vi "Find Center.vi"(5 "Position":i32, 7 "Tray Number":dbl format="%#_13g", 8 "Type of Hexaboard":T1, 9 "XYZTheta":dbl[](array[numeric]), 11 "Gantry In":refnum<k24>) -> (1 "XYZTheta Centers":dbl[][](array[numeric]), 3 "Gantry Out":refnum<k24>)   [LabVIEW 2021, in "Assembly Tray.lvclass"]
uses:
  Assembly Tray.lvclass
  Find Tray.ctl
  Controller/Camera/Machine Vision.ctl
  C:/Program Files (x86)/Aerotech/A3200/LabVIEW/2010/Bin/Aerotech.A3200.dll
  Program Files (x86)/Aerotech/A3200/LabVIEW/2010/Bin/Aerotech.A3200.dll
  Controller/Camera/Image processing.ctl
  Controller/Camera/Camera settings.ctl
  Controller/Camera/Material.ctl
  Routine/TypeOfHexaboard.ctl
  Program Files (x86)/National Instruments/LabVIEW 2021/examples/Connectivity/Python/support/PythonVersionsEnum.ctl
  Controller/Camera/Camera.lvclass
  Controller/Motion/A3200/A3200.lvclass
  Controller/Motion/Motion.lvclass
  Routine/Routine.lvclass
panel:
  out "Move by":dbl[](array[numeric])
  in  "Autofiducial (Beta)":bool
  in  "Focus step size":dbl format="%#_13g"
  in  "number of focus steps":i32
  out "Average Strength":dbl
  in  "Focus":bool
  in  "Material":T2
  in  "Camera settings":T3={"Gamma"=1.6, "Gain"=0, "Sharpness"=0, "Contrast"=0.0, "Exposure"=0.0078125} {"Exposure" min=0.000244140625 max=0.5 scale=0.0002..0.5; "Contrast" min=0.0 max=1.0 scale=0.001..1.0; "Sharpness" min=0 max=2 step=1 scale=0.0..2.0; "Gain" min=0 max=100 step=1 scale=0.1..100.0; "Gamma" min=0.01 max=10.0 scale=0.01..10.0}
  in  "Image processing":T4={"Brightness"=128.0, "Contrast"=45.0, "Gamma"=1.0471123} {"Brightness" scale=0.0..400.0; "Contrast" scale=0.0..90.0; "Gamma" scale=0.005..5.0}
  in  "Override presets":bool
  out "Both fiducials recorded":bool
  in  "Machine Vision":T5
  out "Right Fiducial":dbl[](array[numeric]) format="%.6g"
  out "Left Fiducial":dbl[](array[numeric]) format="%.6g"
  out "Gantry":dbl[](array[numeric]) format="%.6g"
  out "Sum":dbl[](array[numeric]) format="%.6g"
  out "Camera":dbl[](array[numeric]) format="%.6g"
  in  "Carrier Tray":T6
  out "Image":T7(plugin-control)
  out "Center":dbl[](array[numeric]) format="%.6g"
  in  "Position Number":i16
  in  "Go to Center":bool
  in  "Calculate":bool
  in  "Record Bottom":bool
  in  "Record Top":bool
  in  "Go to Bottom Fiducial":bool
  in  "Go to Top Fiducial":bool
  in  "Joystick":bool
  in  "Stop":bool
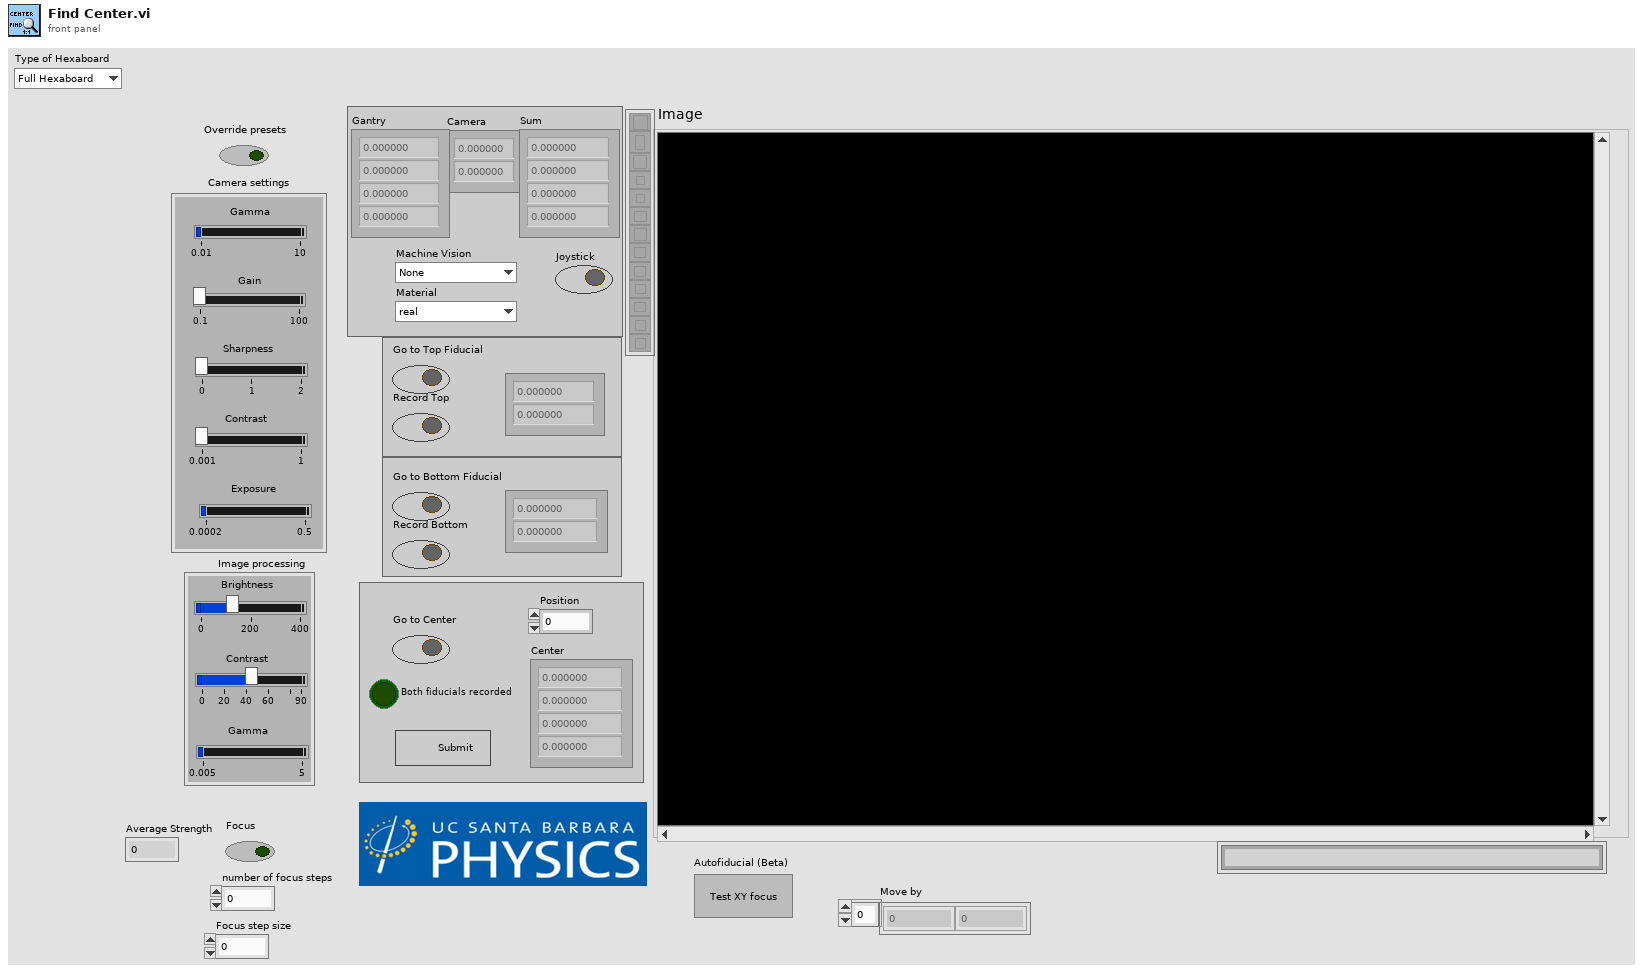
[diagram p1: front panel]
types:
  T1 = typedef "Routine.lvclass/TypeOfHexaboard.ctl" = enum16{"Full Hexaboard", "Right Partial PCB", "Right Partial Sensor", "Al Dummy Right Partial Sensor"}
  T2 = typedef "Camera.lvclass/Material.ctl" = enum16{"real", "dummy", "PETG"}
  T3 = typedef "Camera.lvclass/Camera settings.ctl" = cluster{"Gamma":dbl, "Gain":i64, "Sharpness":i64, "Contrast":dbl, "Exposure":dbl}
  T4 = typedef "Camera.lvclass/Image processing.ctl" = cluster{"Brightness":sgl, "Contrast":sgl, "Gamma":sgl}
  T5 = typedef "Camera.lvclass/Machine Vision.ctl" = enum16{"None", "Tray Fiducials", "Sensor Fiducials", "HPK Silicon", "Partial Hexaboard", "Partial Hexaboard Test", "100um dot", "Hexaboard", "Corner (TL, BR)", "Corner (BL, TR)", "V3 Sensor Cross", "V3 Sensor Circle"}
  T6 = typedef "Assembly Tray.lvclass/Find Tray.ctl" = cluster{"Gantry Fiducials":dbl[], "Relative Coordinates":dbl[][], "Camera Fiducials":dbl[][], "XYZTheta Centers":dbl[][], "Workspace Center":dbl[], "Syringe Relative Coordinates":dbl[], "Gantry Region":dbl, "Fiducials":path, "New Fiducials":dbl[][], "Past Fiducials":dbl[][], "XYZTheta":dbl[], "Position":dbl}
  T7 = typedef "IMAQ Image.ctl" = refnum<image>
  T8 = typedef "PythonVersionsEnum.ctl" = enum16{"3.6", "3.7", "3.8", "3.9"}
  T9 = typedef "File Paths.ctl" = cluster{"Glue Pattern Folder":path, "Carrier Tray Folder":path, "Pick Up Tool Fixture Folder":path, "Components Folder":path, "Bellows Tool Offset.txt":path, "Pick Up Tool Offset.txt":path, "Dispense Tip Offset.txt":path, "Log Files":path, "Gantry Assembly Map.txt":path, "Syringe and offset map.txt":path}
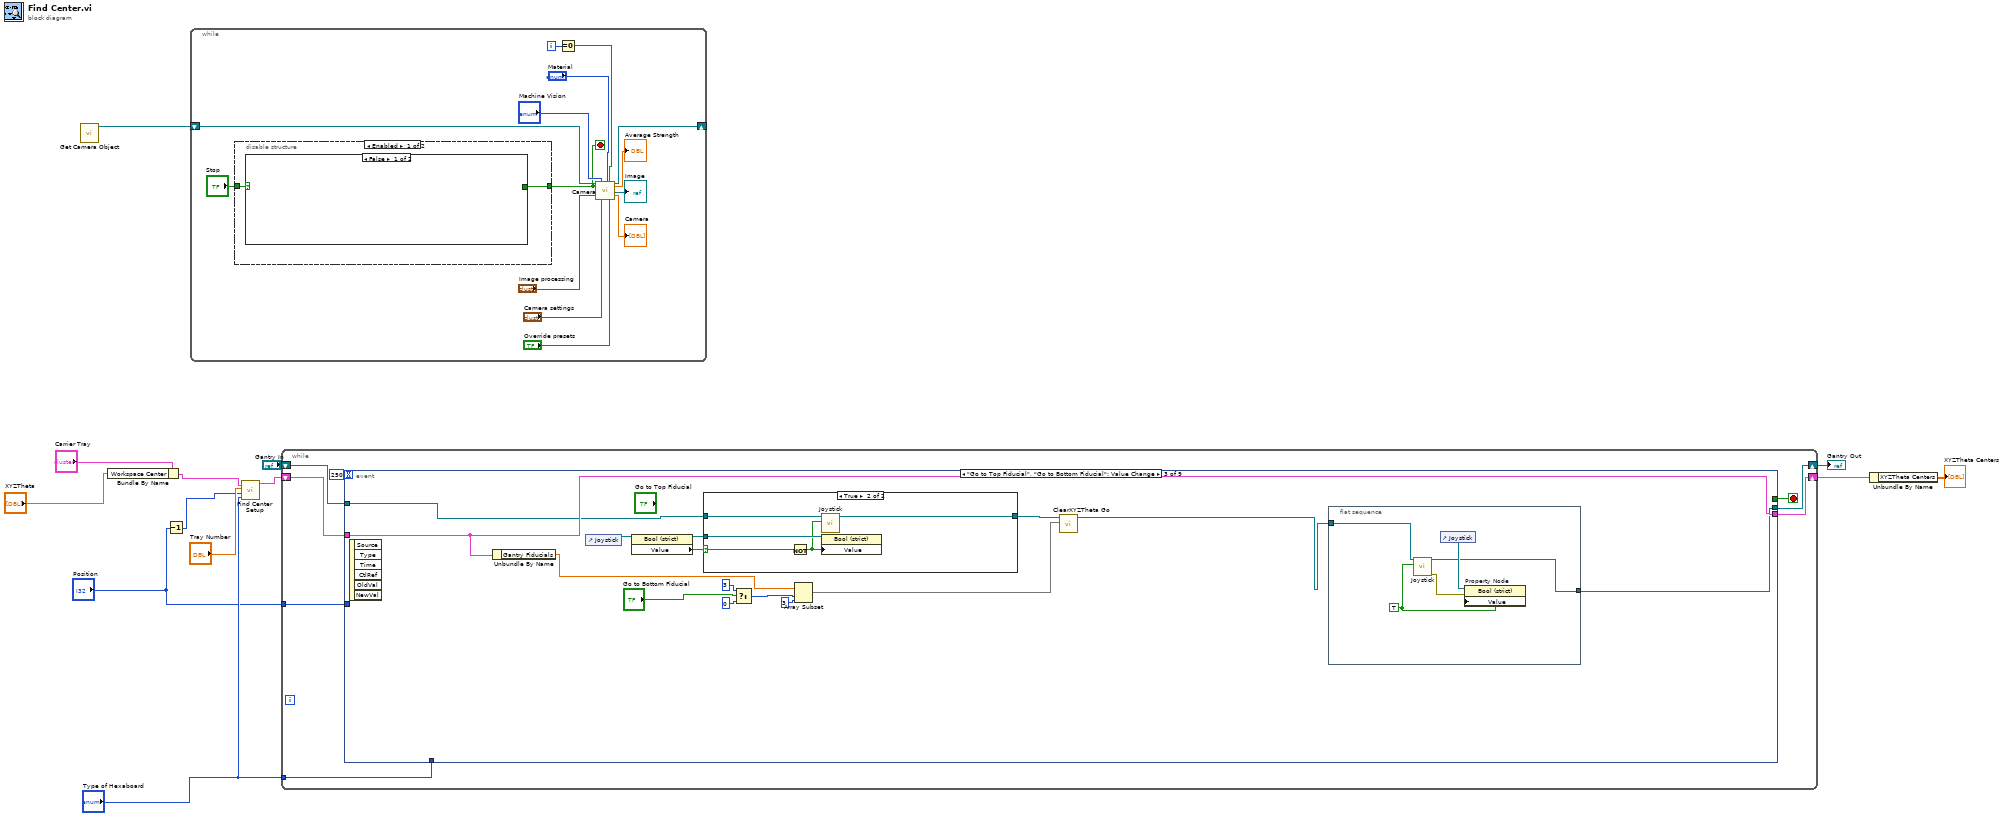
[diagram p0: block diagram]
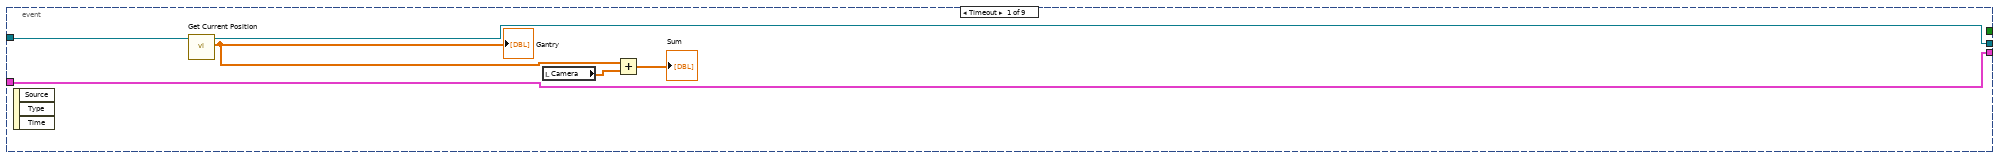
[diagram p2: hidden frame]
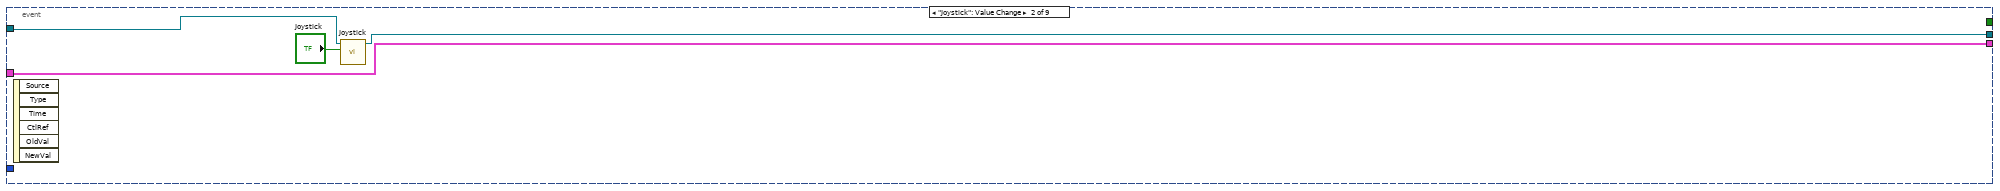
[diagram p3: hidden frame]
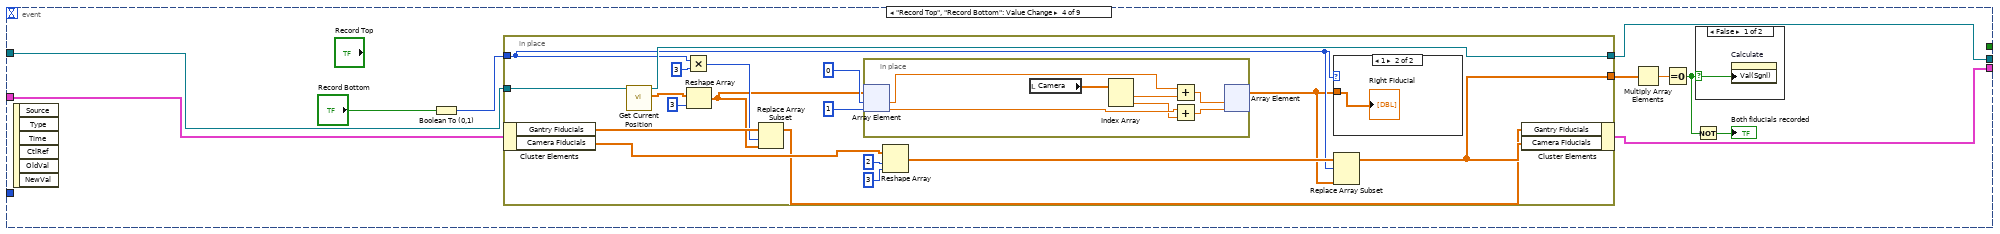
[diagram p5: hidden frame]
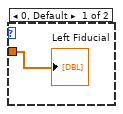
[diagram p7: hidden frame]
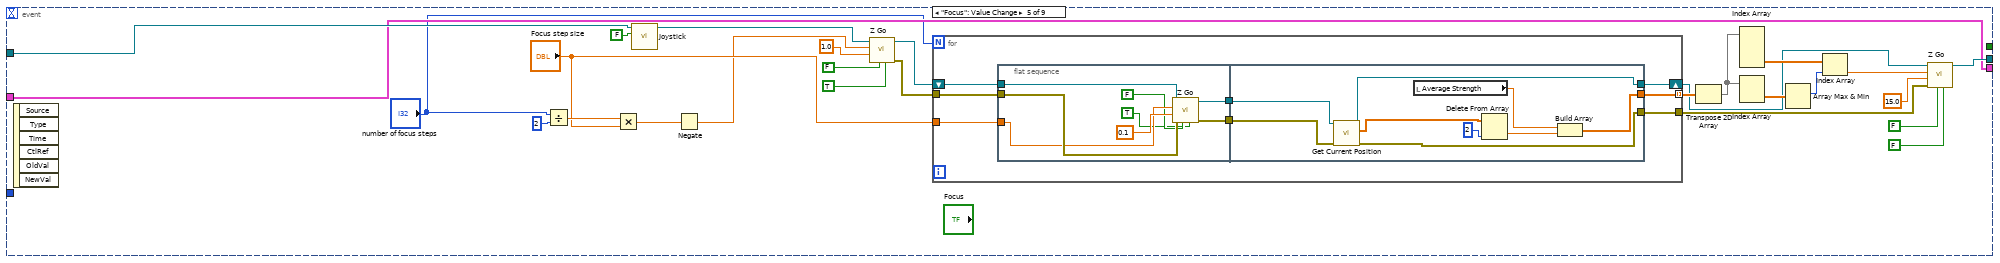
[diagram p8: hidden frame]
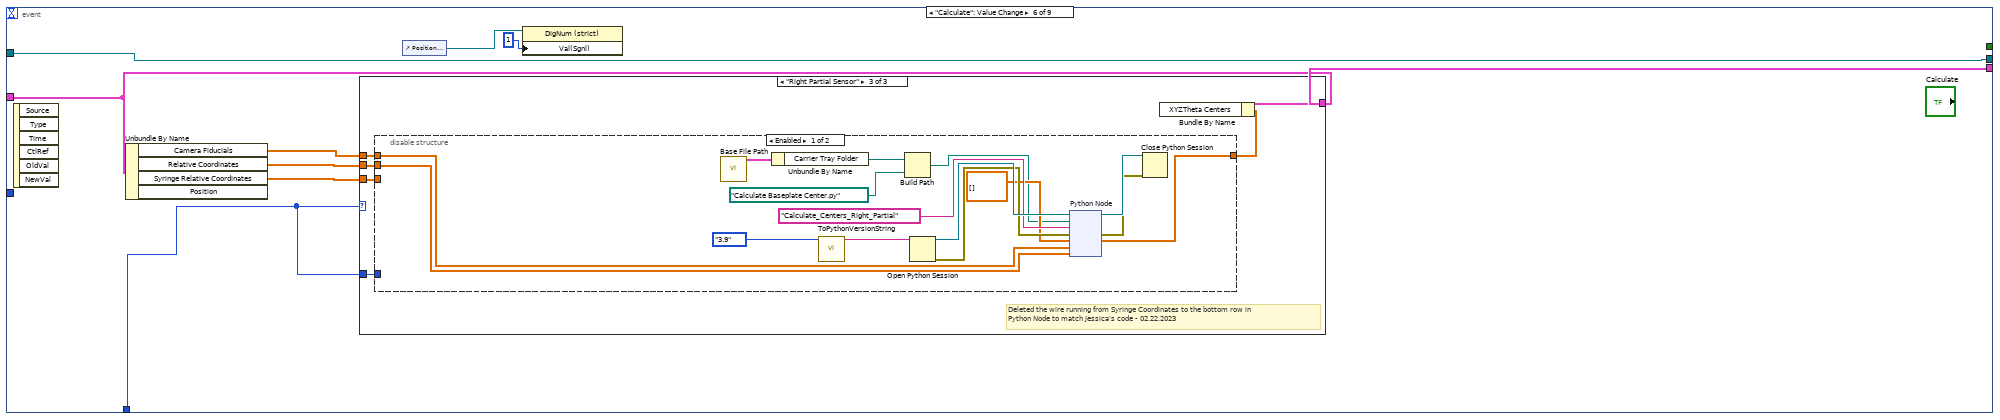
[diagram p9: hidden frame]
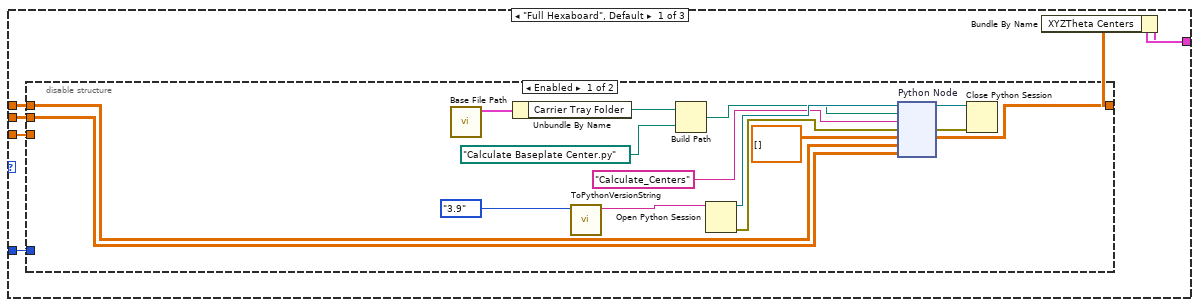
[diagram p10: hidden frame]
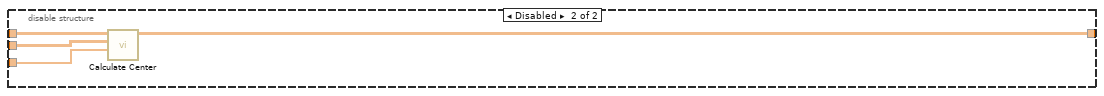
[diagram p11: hidden frame]
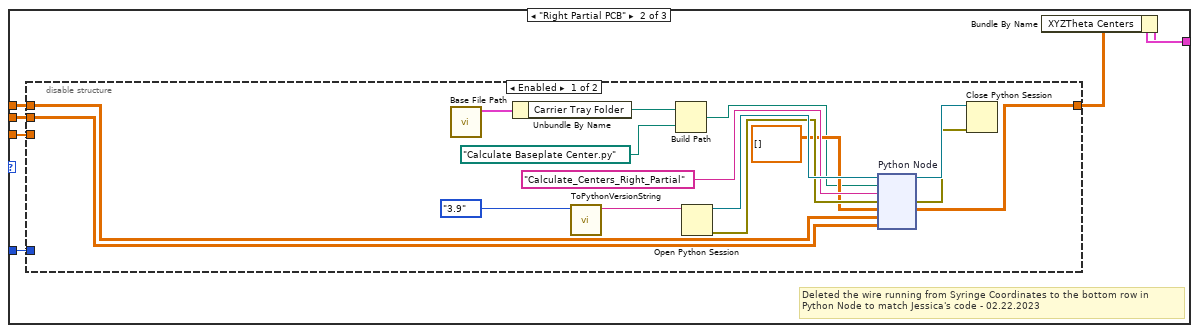
[diagram p12: hidden frame]
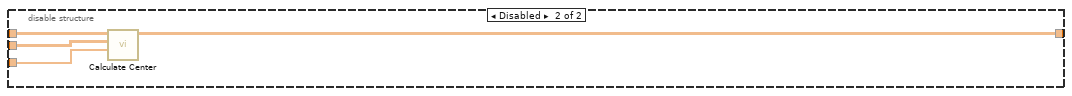
[diagram p13: hidden frame]
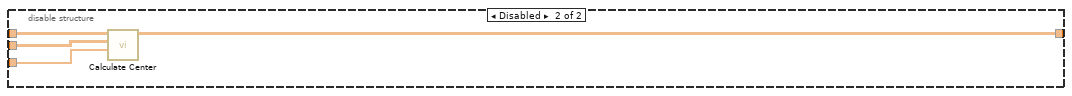
[diagram p14: hidden frame]
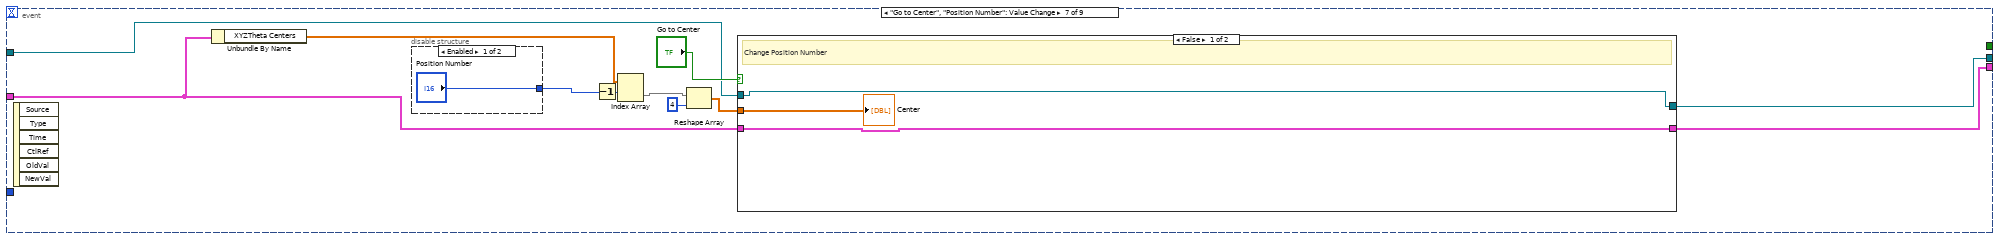
[diagram p15: hidden frame]
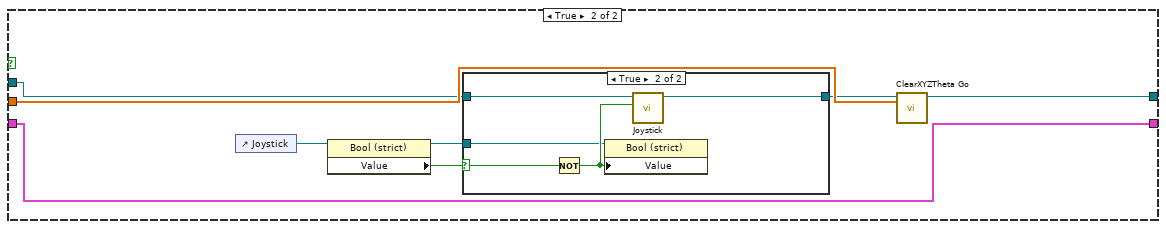
[diagram p17: hidden frame]
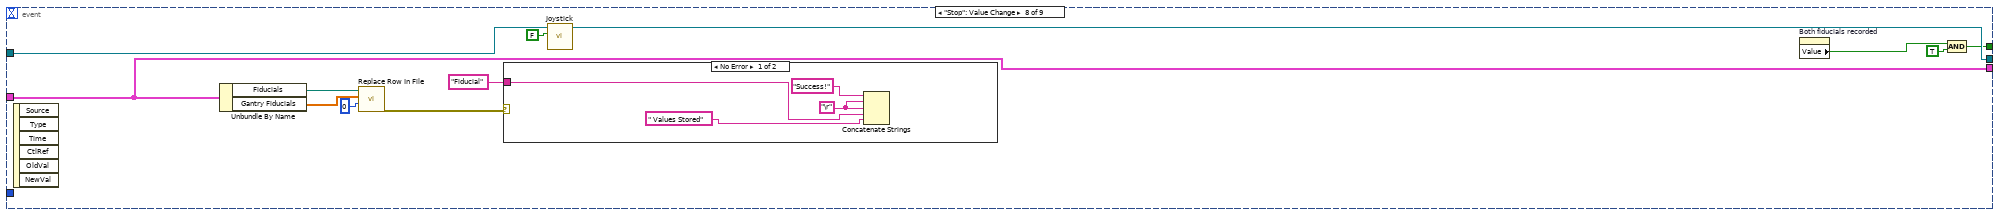
[diagram p19: hidden frame]
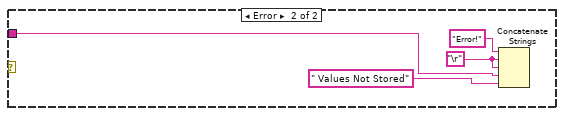
[diagram p20: hidden frame]
diagram:
  n1 = call "Get Camera Object.vi"() -> ("Camera out"=w6:refnum<class "Camera.lvclass">)  [unwired: 10 in, 1 out]
  n2 = Bundle By Name(cluster="Carrier Tray", "Workspace Center"="XYZTheta") -> (w10:T6)
  n3 = Decrement(x="Position") -> (x-1=w3:i32)
  n4 = while {
    shift-right: [w23] -> _
    shift-left: w6 -> [w27]
    i -> [w17]
    stop <- w22 stop-if-true
    n5 = disable-structure shown="Enabled" {
      disable-tunnel: [w28 w35] -> w22
      disable-tunnel: "Stop" -> [w29 w35]
      frame Enabled {
        n6 = case shown="False" w29 {
          tunnel: [_ w30] -> w28
          frame False {
          }
          frame True {
            n7 = property on="Both fiducials recorded" class="Bool (strict)"() -> ("Value"=w31:bool)  [unwired: 2 in, 2 out]
            n8 = case shown="False" w31 {
              tunnel: [_ TRUE] -> w30
              frame False {
                n9 = One Button Dialog(message="Atleast one fiducial not recorded!") -> ()  [unwired: 1 in, 1 out]
              }
              frame True {
                n10 = property on="Both fiducials recorded" class="Bool (strict)"("Val(Sgnl)"=FALSE) -> ()  [unwired: 2 in, 2 out]
              }
            }
          }
        }
      }
      frame Disabled {
      }
    }
    n11 = Equal To 0?(x=w17) -> (x = 0?=w16:bool)
    n12 = call "Camera.vi"("Camera in"=w27, "Stop"=w22, "BCG Image Processing"="Image processing", "Machine Vision"="Machine Vision", "Camera settings"="Camera settings", "Material"="Material", "Loop 0"=w16, "Override presets"="Override presets") -> ("Camera out"=w23:refnum<class "Camera.lvclass">, "Average Strength"=→"Average Strength":dbl, "Image"=→"Image":T7, "Camera"=→"Camera":dbl[])  [unwired: 5 in, 3 out]
  }
  n13 = call "Find Center Setup.vi"("Carrier Tray"=w10, "Tray Number"="Tray Number", "Position"=w3, "Type of Hexaboard"="Type of Hexaboard") -> ("Assembly Tray Out"=w13:T6)  [unwired: 6 in]
  n14 = while {
    shift-right: [w42] -> w12
    shift-left: w13 -> [w43]
    shift-right: [w38] -> w4
    shift-left: "Gantry In" -> [w39]
    tunnel: "Type of Hexaboard" -> [w37]
    tunnel: "Position" -> [w36]
    stop <- w41 stop-if-true
    n15 = event shown="[2] \"Go to Top Fiducial\", \"Go to Bottom Fiducial\": Value Change" {
      selector: _ -> [_ _ _ _ _ _ _ _ _]
      dyn-events: _ -> [_ _ _ _ _ _ _ _ _]
      timeout: 250 -> [_ _ _ _ _ _ _ _ _]
      tunnel: [w47 w53 w68 w89 w129 w176 w266 w293 w306] -> w42
      tunnel: w43 -> [w47 w53 w68 w84 w129 w170 w267 w293 w306]
      tunnel: [_ _ _ _ _ _ _ w288 _] -> w41
      tunnel: w39 -> [w46 w52 w60 w83 w131 w175 w264 w294 w308]
      tunnel: [w44 w50 w55 w82 w130 w175 w260 w289 w309] -> w38
      tunnel: w37 -> [_ _ _ _ _ w171 _ _ _]
      tunnel: w36 -> [_ _ _ _ _ _ _ _ _]
      event Timeout {
        n16 = event-data() -> ()  [unwired: 1 in, 3 out]
        n17 = call "Get Current Position.vi"("Gantry In"=w46) -> ("XYZTheta Out"=w45:dbl[], "Gantry Out"=w44:refnum<k24>)  [unwired: 8 in, 1 out]
        "Gantry" <- w45
        n18 = local read "Camera"() -> (w49:dbl[])
        n19 = Add(x=w45, y=w49) -> (x+y=→"Sum":dbl[])
      }
      event "Joystick": Value Change {
        n20 = event-data() -> ()  [unwired: 1 in, 6 out]
        n21 = call "Joystick.vi"("Joystick"="Joystick", "Gantry In"=w52) -> ("Gantry Out"=w50:refnum<k24>)  [unwired: 8 in, 1 out]
      }
      event "Go to Top Fiducial", "Go to Bottom Fiducial": Value Change {
        n22 = event-data() -> ()  [unwired: 1 in, 6 out]
        n23 = Unbundle By Name "Unbundle By Name"(w68) -> ("Gantry Fiducials"=w57:dbl[])
        n24 = control-ref of="Joystick"() -> (w67:refnum<vi>)
        n25 = property class="Bool (strict)"(reference=w67) -> (reference out=w58:refnum<vi>, "Value"=w61:bool)  [unwired: 1 in, 1 out]
        n26 = case shown="True" w61 {
          selector: w61 -> [_ w79]
          tunnel: w60 -> [w74 w77]
          tunnel: [w74 w76] -> w59
          tunnel: w58 -> [_ w78]
          frame False {
          }
          frame True {
            n27 = Not(x=w79) -> (.not. x?=w75:bool)
            n28 = call "Joystick.vi"("Joystick"=w75, "Gantry In"=w77) -> ("Gantry Out"=w76:refnum<k24>)  [unwired: 8 in, 1 out]
            n29 = property class="Bool (strict)"(reference=w78, "Value"=w75) -> ()  [unwired: 1 in, 2 out]
          }
        }
        n30 = Select(t=3, s="Go to Bottom Fiducial", f=0) -> (s? t:f=w65:i32)
        n31 = Array Subset "Array Subset"(array=w57, index=w65, length=3) -> (w56:dbl[])
        n32 = call "ClearXYZTheta Go.vi"("XYZTheta In"=w56, "Gantry In"=w59) -> ("Gantry Out"=w54:refnum<k24>)  [unwired: 7 in, 2 out]
        n33 = flat-sequence {
          tunnel: w54 -> [w73]
          tunnel: [w70] -> w55
          frame #0 {
            w69 = TRUE
            n34 = call "Joystick.vi"("Joystick"=w69, "Gantry In"=w73) -> ("error out"=w71:errorcluster, "Gantry Out"=w70:refnum<k24>)  [unwired: 8 in]
            n35 = control-ref of="Joystick"() -> (w72:refnum<vi>)
            n36 = property on="Property Node" class="Bool (strict)"(reference=w72, error in=w71, "Value"=w69) -> ()  [unwired: 2 out]
          }
        }
      }
      event "Record Top", "Record Bottom": Value Change {
        n37 = event-data() -> ()  [unwired: 1 in, 6 out]
        n38 = Boolean To (0,1)(Boolean="Record Bottom") -> (0, 1=w86:i16)
        n39 = in-place {
          in-place-border: [w102] -> w87
          in-place-border: w86 -> [w95]
          in-place-border: w83 -> [w97]
          in-place-border: [w96] -> w82
          n40 = in-place-cluster #1(w84) -> ("Gantry Fiducials"=w99:dbl[], "Camera Fiducials"=w106:dbl[][])
          n41 = call "Get Current Position.vi"("Gantry In"=w97) -> ("XYZTheta Out"=w100:dbl[], "Gantry Out"=w96:refnum<k24>)  [unwired: 8 in, 1 out]
          n42 = Multiply(x=w95, y=i16 3) -> (x*y=w93:i16)
          n43 = Reshape Array(w100, 3 ("dimension size")) -> (w92:dbl[])
          n44 = Replace Array Subset(array=w99, new element=w92, index=w93) -> (w98:dbl[])
          n45 = in-place {
            n46 = in-place-array #2(w92, 0, 1) -> (w114:dbl, w112:dbl)
            n47 = local read "Camera"() -> (w115:dbl[])
            n48 = Index Array(array=w115) -> (element #1=w113:dbl, element #2=w111:dbl)  [unwired: 2 in]
            n49 = Add(x=w114, y=w113) -> (x+y=w109:dbl)
            n50 = Add(x=w112, y=w111) -> (x+y=w110:dbl)
            n51 = in-place-array #2(w109, w110) -> (w91:dbl[])  [unwired: 2 out]
          }
          n52 = Reshape Array(w106, 2 ("length"), 3 ("dimension size")) -> (w105:dbl[][])
          n53 = case shown="1" w95 {
            tunnel: w91 -> [w116 w117]
            frame 0, Default {
              "Left Fiducial" <- w116
            }
            frame 1 {
              "Right Fiducial" <- w117
            }
          }
          n54 = Replace Array Subset(array=w105, new element=w91, index (row)=w95) -> (w102:dbl[][])  [unwired: 1 in]
          n55 = in-place-cluster #1("Gantry Fiducials"=w98, "Camera Fiducials"=w102) -> (w89:T6)
        }
        n56 = Multiply Array Elements(1:w87) -> (0:w88:dbl)
        n57 = Equal To 0?(x=w88) -> (x = 0?=w81:bool)
        n58 = Not(x=w81) -> (.not. x?=→"Both fiducials recorded":bool)
        n59 = case shown="False" w81 {
          selector: w81 -> [w90 _]
          frame False {
            n60 = property on="Calculate" class="Bool (strict)"("Val(Sgnl)"=w90) -> ()  [unwired: 2 in, 2 out]
          }
          frame True {
          }
        }
      }
      event "Focus": Value Change {
        n61 = event-data() -> ()  [unwired: 1 in, 6 out]
        n62 = Divide(x="number of focus steps", y=2) -> (x/y=w133:dbl)
        n63 = Multiply(x=w133, y="Focus step size") -> (x*y=w132:dbl)
        n64 = call "Joystick.vi"("Joystick"=FALSE, "Gantry In"=w131) -> ("Gantry Out"=w125:refnum<k24>)  [unwired: 8 in, 1 out]
        n65 = Negate(x=w132) -> (-x=w123:dbl)
        n66 = call "Z Go.vi"("Increment"=TRUE, "Return Immediately"=FALSE ("Increment"), "Speed In"=1.0 ("Speed"), "Position In"=w123, "Gantry In"=w125) -> ("error out"=w120:errorcluster, "Gantry Out"=w124:refnum<k24>)  [unwired: 3 in, 2 out]
        n67 = for {
          N: "number of focus steps" -> [_]
          tunnel: [w149] -> w143 mode=indexing
          tunnel: w120 -> [w148]
          tunnel: [w146] -> w136
          shift-right: [w150] -> w137
          shift-left: w124 -> [w152]
          tunnel: "Focus step size" -> [w145]
          n68 = flat-sequence {
            tunnel: w152 -> [w160]
            tunnel: [w159] -> w151
            tunnel: w148 -> [w157]
            tunnel: [w158] -> w147
            tunnel: w145 -> [w155]
            tunnel: w151 -> [w169]
            tunnel: [w168] -> w150
            tunnel: [w167] -> w149
            tunnel: w147 -> [w163]
            tunnel: [w162] -> w146
            frame #0 {
              n69 = call "Z Go.vi"("Increment"=TRUE, "Return Immediately"=FALSE ("Increment"), "error in (no error)"=w157, "Speed In"=0.1 ("Speed"), "Position In"=w155, "Gantry In"=w160) -> ("error out"=w158:errorcluster, "Gantry Out"=w159:refnum<k24>)  [unwired: 2 in, 2 out]
            }
            frame #1 {
              n70 = call "Get Current Position.vi"("error in (no error)"=w163, "Gantry In"=w169) -> ("error out"=w162:errorcluster, "XYZTheta Out"=w166:dbl[], "Gantry Out"=w168:refnum<k24>)  [unwired: 7 in]
              n71 = local read "Average Strength"() -> (w161:dbl)
              n72 = Delete From Array(array=w166, index=2) -> (deleted portion=w164:dbl)  [unwired: 1 in, 1 out]
              n73 = Build Array(w161, w164) -> (w167:dbl[])
            }
          }
        }
        n74 = Transpose 2D Array(2D array=w143) -> (transposed array=w142:dbl[][])
        n75 = Index Array(array=w142) -> (element #2=w141:dbl[])  [unwired: 4 in, 1 out]
        n76 = Index Array(array=w142) -> (element=w144:dbl[])  [unwired: 2 in]
        n77 = Array Max & Min(array=w144) -> (max index (indices)=w140:i32)  [unwired: 3 out]
        n78 = Index Array(array=w141, index=w140) -> (element=w139:dbl)
        n79 = call "Z Go.vi"("Increment"=FALSE, "Return Immediately"=FALSE ("Increment"), "error in (no error)"=w136, "Speed In"=15.0 ("Speed"), "Position In"=w139, "Gantry In"=w137) -> ("Gantry Out"=w130:refnum<k24>)  [unwired: 2 in, 3 out]
      }
      event "Calculate": Value Change {
        n80 = event-data() -> ()  [unwired: 1 in, 6 out]
        n81 = Unbundle By Name "Unbundle By Name"(w170) -> ("Camera Fiducials"=w172:dbl[][], "Relative Coordinates"=w173:dbl[][], "Syringe Relative Coordinates"=w174:dbl[])  [unwired: 1 out]
        n82 = case shown="\"Right Partial Sensor\"" w171 {
          tunnel: w170 -> [w185 w211 w237]
          tunnel: [w184 w210 w236] -> w176
          tunnel: w174 -> [w183 w209 w235]
          tunnel: w173 -> [w182 w208 w234]
          tunnel: w172 -> [w181 w207 w233]
          tunnel: w171 -> [w179 w205 w231]
          frame "Full Hexaboard", Default {
            n83 = disable-structure shown="Enabled" {
              disable-tunnel: w181 -> [w192 w203]
              disable-tunnel: w182 -> [w191 w202]
              disable-tunnel: w183 -> [_ w201]
              disable-tunnel: [w186 w204] -> w180
              disable-tunnel: w179 -> [_ _]
              frame Enabled {
                n84 = call "Base File Path.vi"() -> ("Paths Out"=w193:T9)  [unwired: 11 in]
                n85 = Unbundle By Name(w193) -> ("Carrier Tray Folder"=w189:path)
                n86 = call "ToPythonVersionString.vi"("python version"=PythonVersionsEnum."3.9") -> ("python version string"=w199:string)  [unwired: 10 in]
                n87 = Build Path(base path=w189, name or relative path=path "Calculate Baseplate Center.py") -> (appended path=w188:path)
                n88 = Open Python Session(python version=w199) -> (session out=w198:refnum<k35>, error out=w196:errorcluster)  [unwired: 2 in]
                n89 = node "Python Node"(w198, w188, "Calculate_Centers" ("function name"), w196, dbl[][] [], w192, w191) -> (w197:refnum<k35>, w195:errorcluster, w186:dbl[][])  [unwired: 2 in, 2 out]
                n90 = Close Python Session(session in=w197, error in=w195) -> ()  [unwired: 1 out]
              }
              frame Disabled {
                n91 = call "Calculate Center.vi"("Syringe Coordinates"=w201, "Relative Coordinates"=w202, "Fiducial Measurements"=w203) -> ("XYZTheta Centers"=w204:dbl[][])  [unwired: 8 in]
              }
            }
            n92 = Bundle By Name(cluster=w185, "XYZTheta Centers"=w180) -> (w184:T6)
          }
          frame "Right Partial PCB" {
            # "Deleted the wire running from Syringe Coordinates to the bottom row in\nPython Node to match Jessica's code - 02.22.2023"
            n93 = disable-structure shown="Enabled" {
              disable-tunnel: w207 -> [w218 w229]
              disable-tunnel: w208 -> [w217 w228]
              disable-tunnel: w209 -> [_ w227]
              disable-tunnel: [w212 w230] -> w206
              disable-tunnel: w205 -> [_ _]
              frame Enabled {
                n94 = call "Base File Path.vi"() -> ("Paths Out"=w219:T9)  [unwired: 11 in]
                n95 = Unbundle By Name(w219) -> ("Carrier Tray Folder"=w215:path)
                n96 = call "ToPythonVersionString.vi"("python version"=PythonVersionsEnum."3.9") -> ("python version string"=w225:string)  [unwired: 10 in]
                n97 = Build Path(base path=w215, name or relative path=path "Calculate Baseplate Center.py") -> (appended path=w214:path)
                n98 = Open Python Session(python version=w225) -> (session out=w224:refnum<k35>, error out=w222:errorcluster)  [unwired: 2 in]
                n99 = node "Python Node"(w224, w214, "Calculate_Centers_Right_Partial" ("function name"), w222, dbl[][] [], w218, w217) -> (w223:refnum<k35>, w221:errorcluster, w212:dbl[][])  [unwired: 2 in, 2 out]
                n100 = Close Python Session(session in=w223, error in=w221) -> ()  [unwired: 1 out]
              }
              frame Disabled {
                n101 = call "Calculate Center.vi"("Syringe Coordinates"=w227, "Relative Coordinates"=w228, "Fiducial Measurements"=w229) -> ("XYZTheta Centers"=w230:dbl[][])  [unwired: 8 in]
              }
            }
            n102 = Bundle By Name(cluster=w211, "XYZTheta Centers"=w206) -> (w210:T6)
          }
          frame "Right Partial Sensor" {
            # "Deleted the wire running from Syringe Coordinates to the bottom row in\nPython Node to match Jessica's code - 02.22.2023"
            n103 = disable-structure shown="Enabled" {
              disable-tunnel: w233 -> [w244 w255]
              disable-tunnel: w234 -> [w243 w254]
              disable-tunnel: w235 -> [_ w253]
              disable-tunnel: [w238 w256] -> w232
              disable-tunnel: w231 -> [_ _]
              frame Enabled {
                n104 = call "Base File Path.vi"() -> ("Paths Out"=w245:T9)  [unwired: 11 in]
                n105 = Unbundle By Name(w245) -> ("Carrier Tray Folder"=w241:path)
                n106 = call "ToPythonVersionString.vi"("python version"=PythonVersionsEnum."3.9") -> ("python version string"=w251:string)  [unwired: 10 in]
                n107 = Build Path(base path=w241, name or relative path=path "Calculate Baseplate Center.py") -> (appended path=w240:path)
                n108 = Open Python Session(python version=w251) -> (session out=w250:refnum<k35>, error out=w248:errorcluster)  [unwired: 2 in]
                n109 = node "Python Node"(w250, w240, "Calculate_Centers_Right_Partial" ("function name"), w248, dbl[][] [], w244, w243) -> (w249:refnum<k35>, w247:errorcluster, w238:dbl[][])  [unwired: 2 in, 2 out]
                n110 = Close Python Session(session in=w249, error in=w247) -> ()  [unwired: 1 out]
              }
              frame Disabled {
                n111 = call "Calculate Center.vi"("Syringe Coordinates"=w253, "Relative Coordinates"=w254, "Fiducial Measurements"=w255) -> ("XYZTheta Centers"=w256:dbl[][])  [unwired: 8 in]
              }
            }
            n112 = Bundle By Name(cluster=w237, "XYZTheta Centers"=w232) -> (w236:T6)
          }
        }
        n113 = control-ref of="Position Number"() -> (w178:refnum<vi>)
        n114 = property class="DigNum (strict)"(reference=w178, "Val(Sgnl)"=i16 1 ("Value (Signaling)")) -> ()  [unwired: 1 in, 2 out]
      }
      event "Go to Center", "Position Number": Value Change {
        n115 = event-data() -> ()  [unwired: 1 in, 6 out]
        n116 = Unbundle By Name(w267) -> ("XYZTheta Centers"=w259:dbl[][])
        n117 = disable-structure shown="Enabled" {
          disable-tunnel: ["Position Number" _] -> w257
          frame Enabled {
          }
          frame Disabled {
          }
        }
        n118 = Decrement(x=w257) -> (x-1=w258:i16)
        n119 = Index Array "Index Array"(array=w259, index (row)=w258) -> (element=w262:dbl[])  [unwired: 1 in]
        n120 = Reshape Array "Reshape Array"(w262, u32 4) -> (w261:dbl[])
        n121 = case shown="False" "Go to Center" {
          tunnel: w261 -> [w271 w277]
          tunnel: w267 -> [w270 w279]
          tunnel: [w270 w279] -> w266
          tunnel: w264 -> [w269 w273]
          tunnel: [w269 w278] -> w260
          frame False {
            # "Change Position Number"
            "Center" <- w271
          }
          frame True {
            n122 = control-ref of="Joystick"() -> (w276:refnum<vi>)
            n123 = property class="Bool (strict)"(reference=w276) -> (reference out=w274:refnum<vi>, "Value"=w275:bool)  [unwired: 1 in, 1 out]
            n124 = case shown="True" w275 {
              selector: w275 -> [_ w285]
              tunnel: w273 -> [w280 w284]
              tunnel: [w280 w283] -> w272
              tunnel: w274 -> [_ w281]
              frame False {
              }
              frame True {
                n125 = Not(x=w285) -> (.not. x?=w282:bool)
                n126 = property class="Bool (strict)"(reference=w281, "Value"=w282) -> ()  [unwired: 1 in, 2 out]
                n127 = call "Joystick.vi"("Joystick"=w282, "Gantry In"=w284) -> ("Gantry Out"=w283:refnum<k24>)  [unwired: 8 in, 1 out]
              }
            }
            n128 = call "ClearXYZTheta Go.vi"("XYZTheta In"=w277, "Gantry In"=w272) -> ("Gantry Out"=w278:refnum<k24>)  [unwired: 7 in, 2 out]
          }
        }
      }
      event "Stop": Value Change {
        n129 = event-data() -> ()  [unwired: 1 in, 6 out]
        n130 = Unbundle By Name(w293) -> ("Fiducials"=w291:path, "Gantry Fiducials"=w292:dbl[])
        n131 = call "Replace Row In File.vi"("Index"=0, "Insert Array"=w292, "Path"=w291) -> ("error out"=w297:errorcluster)  [unwired: 8 in]
        n132 = case shown="No Error" w297 {
          tunnel: "Fiducial" -> [w298 w305]
          frame No Error {
            w299 = "\r"
            n133 = Concatenate Strings("Success!", w299, w299, w298, " Values Stored") -> ()  [unwired: 1 out]
          }
          frame Error {
            w302 = "\r"
            n134 = Concatenate Strings("Error!", w302, w302, w305, " Values Not Stored") -> ()  [unwired: 1 out]
          }
        }
        n135 = call "Joystick.vi"("Joystick"=FALSE, "Gantry In"=w294) -> ("Gantry Out"=w289:refnum<k24>)  [unwired: 8 in, 1 out]
        n136 = property on="Both fiducials recorded" class="Bool (strict)"() -> ("Value"=w286:bool)  [unwired: 2 in, 2 out]
        n137 = And(x=w286, y=TRUE) -> (x .and. y?=w288:bool)
      }
      event "Autofiducial (Beta)": Value Change {
        n138 = event-data() -> ()  [unwired: 1 in, 6 out]
        n139 = disable-structure shown="Enabled" {
          disable-tunnel: [w313 w340] -> w309
          disable-tunnel: w308 -> [w312 w340]
          disable-tunnel: "Autofiducial (Beta)" -> [w311 _]
          frame Enabled {
            n140 = flat-sequence {
              tunnel: w311 -> [_]
              tunnel: [w319] -> w310
              tunnel: w312 -> [w324]
              tunnel: [w324] -> w318
              tunnel: [w323] -> w317
              tunnel: [w322] -> w316
              tunnel: w310 -> [w321]
              tunnel: w318 -> [w328]
              tunnel: [w327] -> w315
              tunnel: w317 -> [w326]
              tunnel: [w325] -> w314
              tunnel: w316 -> [w325]
              tunnel: [w334] -> w313
              tunnel: w315 -> [w335]
              tunnel: w314 -> [w333]
              frame #0 {
                n141 = local read "Image"() -> (w320:T7)
                n142 = call "Find Fiducial.vi"("Image"=w320) -> ("Move by (mm)"=w319:dbl[])  [unwired: 3 in]
              }
              frame #1 {
                n143 = Index Array(array=w321) -> (element #1=w323:dbl, element #2=w322:dbl)  [unwired: 2 in]
                "Move by" <- w321
              }
              frame #2 {
                n144 = call "Joystick.vi"("Joystick"=FALSE, "Gantry In"=w328) -> ("Gantry Out"=w329:refnum<k24>)  [unwired: 8 in, 1 out]
                n145 = call "Move Inc.vi"("Axis"="X", "Speed"=25.0, "Distance"=w326, "Gantry In"=w329) -> ("Gantry Out"=w327:refnum<k24>)  [unwired: 6 in, 1 out]
              }
              frame #3 {
                n146 = call "Joystick.vi"("Joystick"=FALSE, "Gantry In"=w335) -> ("Gantry Out"=w336:refnum<k24>)  [unwired: 8 in, 1 out]
                n147 = call "Move Inc.vi"("Axis"="Y", "Speed"=25.0, "Distance"=w333, "Gantry In"=w336) -> ("Gantry Out"=w334:refnum<k24>)  [unwired: 6 in, 1 out]
              }
            }
          }
          frame Disabled {
          }
        }
      }
    }
  }
  "Gantry Out" <- w4
  n148 = Unbundle By Name(w12) -> ("XYZTheta Centers"=→"XYZTheta Centers":dbl[][])
